vi "CRYSet SoundCard Front Panel.vi"(11 "Vi Ref in":refnum<vi> caption="Vi Ref") -> (3 "Vi Ref out":refnum<vi> caption="Vi Ref")   [LabVIEW 2013]
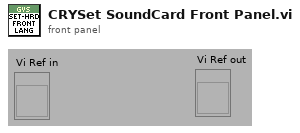
[diagram p1: front panel]
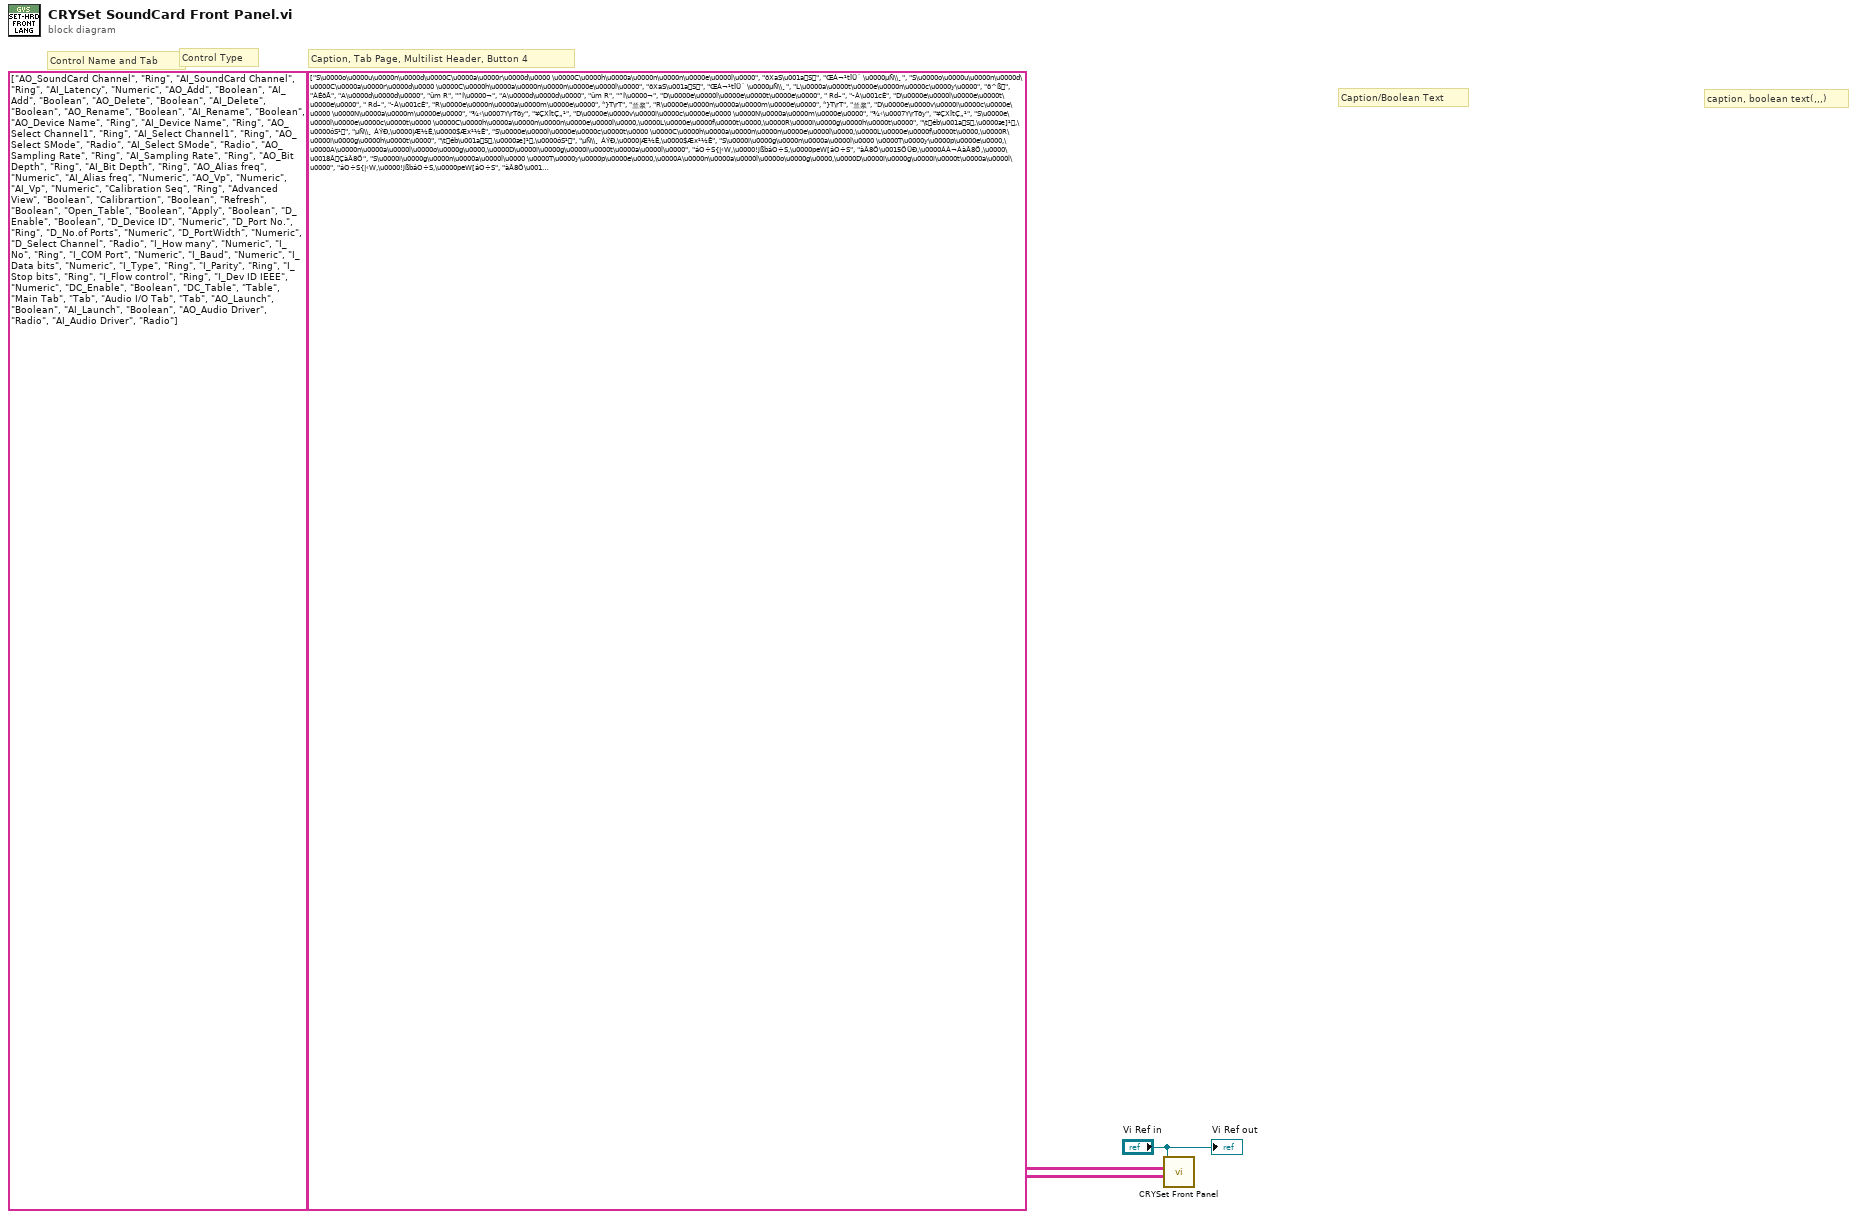
[diagram p0: block diagram]
diagram:
  # "Caption, Tab Page, Multilist Header, Button 4"
  # "Control Type"
  # "Control Name and Tab"
  # "caption, boolean text(,,,)"
  # "Caption/Boolean Text"
  n1 = call "CRYSet Front Panel.vi"("Caption(Boolean Text)"=string[][] [["S\u0000o\u0000u\u0000n\u0000d\u0000C\u0000a\u0000r\u0000d\u0000 \u0000C\u0000h\u0000a\u0000n\u0000n\u0000e\u0000l\u0000", "ðXaS\u001aS", "ŒÁ¬¹tÎÜ´ \u0000µÑ\\¸"], ["S\u0000o\u0000u\u0000n\u0000d\u0000C\u0000a\u0000r\u0000d\u0000 \u0000C\u0000h\u0000a\u0000n\u0000n\u0000e\u0000l\u0000", "ðXaS\u001aS", "ŒÁ¬¹tÎÜ´ \u0000µÑ\\¸"], ["L\u0000a\u0000t\u0000e\u0000n\u0000c\u0000y\u0000", "ö^ß", "ÀÉðÅ"], ["A\u0000d\u0000d\u0000", "ûm R", "”Í\u0000¬"], ["A\u0000d\u0000d\u0000", "ûm R", "”Í\u0000¬"], ["D\u0000e\u0000l\u0000e\u0000t\u0000e\u0000", " Rd–", "­À\u001cÈ"], ["D\u0000e\u0000l\u0000e\u0000t\u0000e\u0000", " Rd–", "­À\u001cÈ"], ["R\u0000e\u0000n\u0000a\u0000m\u0000e\u0000", "͑}T\rT", "兰浆"], ["R\u0000e\u0000n\u0000a\u0000m\u0000e\u0000", "͑}T\rT", "兰浆"], ["D\u0000e\u0000v\u0000i\u0000c\u0000e\u0000 \u0000N\u0000a\u0000m\u0000e\u0000", "¾‹\u0007Y\rTðy", "¥ÇXÎtÇ„¹"], ["D\u0000e\u0000v\u0000i\u0000c\u0000e\u0000 \u0000N\u0000a\u0000m\u0000e\u0000", "¾‹\u0007Y\rTðy", "¥ÇXÎtÇ„¹"], ["S\u0000e\u0000l\u0000e\u0000c\u0000t\u0000 \u0000C\u0000h\u0000a\u0000n\u0000n\u0000e\u0000l\u0000,\u0000L\u0000e\u0000f\u0000t\u0000,\u0000R\u0000i\u0000g\u0000h\u0000t\u0000", "\téb\u001aS,\u0000æ]¹,\u0000óS¹", "µÑ\\¸ ÁÝÐ,\u0000|Æ½Ê,\u0000$Æx¹½Ê"], ["S\u0000e\u0000l\u0000e\u0000c\u0000t\u0000 \u0000C\u0000h\u0000a\u0000n\u0000n\u0000e\u0000l\u0000,\u0000L\u0000e\u0000f\u0000t\u0000,\u0000R\u0000i\u0000g\u0000h\u0000t\u0000", "\téb\u001aS,\u0000æ]¹,\u0000óS¹", "µÑ\\¸ ÁÝÐ,\u0000|Æ½Ê,\u0000$Æx¹½Ê"], ["S\u0000i\u0000g\u0000n\u0000a\u0000l\u0000 \u0000T\u0000y\u0000p\u0000e\u0000,\u0000A\u0000n\u0000a\u0000l\u0000o\u0000g\u0000,\u0000D\u0000i\u0000g\u0000i\u0000t\u0000a\u0000l\u0000", "áO÷S{|‹W,\u0000!jßbáO÷S,\u0000peW[áO÷S", "àÂ8Ö\u0015ÖÜÐ,\u0000ÁÀ¬ÀàÂ8Ö,\u0000\u0018ÂÇàÂ8Ö"], ["S\u0000i\u0000g\u0000n\u0000a\u0000l\u0000 \u0000T\u0000y\u0000p\u0000e\u0000,\u0000A\u0000n\u0000a\u0000l\u0000o\u0000g\u0000,\u0000D\u0000i\u0000g\u0000i\u0000t\u0000a\u0000l\u0000", "áO÷S{|‹W,\u0000!jßbáO÷S,\u0000peW[áO÷S", "àÂ8Ö\u0015ÖÜÐ,\u0000ÁÀ¬ÀàÂ8Ö,\u0000\u0018ÂÇàÂ8Ö"], ["S\u0000a\u0000m\u0000p\u0000l\u0000i\u0000n\u0000g\u0000 \u0000R\u0000a\u0000t\u0000e\u0000", "Ç‘7h‡s", "\\Ôø¼TÖüÈ\fÓ\u0018Â"], ["S\u0000a\u0000m\u0000p\u0000l\u0000i\u0000n\u0000g\u0000 \u0000R\u0000a\u0000t\u0000e\u0000", "Ç‘7h‡s", "\\Ôø¼TÖüÈ\fÓ\u0018Â"], ["B\u0000i\u0000t\u0000 \u0000D\u0000e\u0000p\u0000t\u0000h\u0000", "Ôkyrpe", "É·ÇTÖD¾¸Ò\u0018Â"], ["B\u0000i\u0000t\u0000 \u0000D\u0000e\u0000p\u0000t\u0000h\u0000", "Ôkyrpe", "É·ÇTÖD¾¸Ò\u0018Â"], ["A\u0000l\u0000i\u0000a\u0000s\u0000 \u0000F\u0000r\u0000e\u0000e\u0000 \u0000F\u0000r\u0000e\u0000q\u0000(\u0000H\u0000z\u0000)\u0000", "\u0006Rgs\nNP", "ÈÕ\u0004ÇüÈ\fÓ\u0018Â"], ["A\u0000l\u0000i\u0000a\u0000s\u0000 \u0000F\u0000r\u0000e\u0000e\u0000 \u0000F\u0000r\u0000e\u0000q\u0000(\u0000H\u0000z\u0000)\u0000", "\u0006Rgs\nNP", "ÈÕ\u0004ÇüÈ\fÓ\u0018Â"], ["V\u0000p\u0000", "ð\\<P5u‹S\bÿV\u0000p\u0000\tÿ", "\u0004ÈUÅ(\u0000V\u0000p\u0000)\u0000"], ["V\u0000p\u0000", "ð\\<P5u‹S\bÿV\u0000p\u0000\tÿ", "\u0004ÈUÅ(\u0000V\u0000p\u0000)\u0000"], ["C\u0000a\u0000l\u0000i\u0000b\u0000r\u0000a\u0000t\u0000i\u0000o\u0000n\u0000 \u0000S\u0000e\u0000q\u0000u\u0000e\u0000n\u0000c\u0000e\u0000", "!hÆQ^\u0017R", "P­\u0000Éü¬\u001cÈ,¸"], ["A\u0000d\u0000v\u0000a\u0000n\u0000c\u0000e\u0000d\u0000 \u0000V\u0000i\u0000e\u0000w\u0000", "Ø§~\ty", "Ç8Á× \u0000ô¼0®"], ["C\u0000a\u0000l\u0000i\u0000b\u0000r\u0000a\u0000t\u0000i\u0000o\u0000n\u0000", "!hÆQ", "P­\u0000É"], ["R\u0000e\u0000f\u0000r\u0000e\u0000s\u0000h\u0000", "7R°elxöN", "¥ÇXÎ\u0015Èô¼ \u00001¬àÂ"], ["O\u0000p\u0000e\u0000n\u0000 \u0000T\u0000a\u0000b\u0000l\u0000e\u0000", "Sb\u0000_\u0017Rhˆ", "µÑ\\¸©º]¸"], ["A\u0000p\u0000p\u0000l\u0000y\u0000", "”^(u", "\u0001È©Æ"], ["E\u0000n\u0000a\u0000b\u0000l\u0000e\u0000", "/T(u", "\u0000¬¥²"], ["D\u0000e\u0000v\u0000i\u0000c\u0000e\u0000 \u0000I\u0000D\u0000", "¾‹\u0007Y\u0016÷S", "¥ÇXÎÝÂÄ¼ˆ¼8Ö\u0000"], ["P\u0000o\u0000r\u0000t\u0000 \u0000N\u0000o\u0000.\u0000", "ïzãS\u0016÷S", "ìÓl­ˆ¼8Ö"], ["N\u0000o\u0000.\u0000o\u0000f\u0000 \u0000P\u0000o\u0000r\u0000t\u0000s\u0000", "ïzãSpeÏ‘", "ìÓl­\u001c¬\u0018Â"], ["P\u0000o\u0000r\u0000t\u0000 \u0000W\u0000i\u0000d\u0000t\u0000h\u0000", "ïzãS½[¦^", "ìÓl­íÓ"], ["S\u0000e\u0000l\u0000e\u0000c\u0000t\u0000 \u0000C\u0000h\u0000a\u0000n\u0000n\u0000e\u0000l\u0000,\u0000O\u0000u\u0000t\u0000p\u0000u\u0000t\u0000,\u0000I\u0000n\u0000p\u0000u\u0000t\u0000", "\téb\u001aS,\u0000úQ,\u0000eQ", "µÑ\\¸ ÁÝÐ,\u0000œÍl­,\u0000…Çl­"], ["H\u0000o\u0000w\u0000 \u0000m\u0000a\u0000n\u0000y\u0000?\u0000", "¥cãSpeÏ‘", "‡º\u001c¬…ÇÈ²L®?\u0000"], ["I\u0000n\u0000t\u0000e\u0000r\u0000f\u0000a\u0000c\u0000e\u0000.\u0000N\u0000o", "¥cãS÷S", "\u0000³tºˆ¼8Ö"], ["C\u0000O\u0000M\u0000 \u0000P\u0000o\u0000r\u0000t\u0000", "2NL\u001a¯ïzãS", "C\u0000O\u0000M\u0000ìÓl­"], ["B\u0000a\u0000u\u0000d\u0000 \u0000R\u0000a\u0000t\u0000e\u0000", "âlyr‡s", "ô¼Ü´ÁÄ³"], ["D\u0000a\u0000t\u0000a\u0000 \u0000b\u0000i\u0000t\u0000s\u0000", "pencMO", "ÇÌ¸D¾¸Ò\u0018Â"], ["T\u0000y\u0000p\u0000e\u0000", "{|‹W", "\u0015Ö"], ["P\u0000a\u0000r\u0000i\u0000t\u0000y\u0000", "GYvP'`", "0®°Æ1Á"], ["S\u0000t\u0000o\u0000p\u0000 \u0000b\u0000i\u0000t\u0000s\u0000", "\\PbkMO", "\u0015ÈÀÉD¾¸Ò"], ["F\u0000l\u0000o\u0000w\u0000 \u0000c\u0000o\u0000n\u0000t\u0000r\u0000o\u0000l\u0000", "Am§c6R", "ÇÌ¸P×¹pÈÈ"], ["D\u0000e\u0000v\u0000 \u0000I\u0000D\u0000 \u0000I\u0000E\u0000E\u0000E\u0000", "緥\u0007Y\u0007h茓 \u0000I\u0000E\u0000E\u0000E\u0000", "¥ÇXÎˆ¼8Ö \u0000I\u0000E\u0000E\u0000E\u0000"], ["E\u0000n\u0000a\u0000b\u0000l\u0000e\u0000", "Oý€", "\u0000¬¥²"], ["T\u0000a\u0000b\u0000l\u0000e\u0000", "hˆ", "\\Ô"], ["S\u0000o\u0000u\u0000n\u0000d\u0000C\u0000a\u0000r\u0000d\u0000,\u0000D\u0000i\u0000g\u0000i\u0000t\u0000a\u0000l\u0000 \u0000I\u0000/\u0000O\u0000,\u0000I\u0000n\u0000t\u0000e\u0000r\u0000f\u0000a\u0000c\u0000e\u0000,\u0000H\u0000e\u0000l\u0000p\u0000", "ðXaS,\u0000peW[ \u0000I\u0000/\u0000O\u0000,\u0000¥cãS,\u0000.^©R \u0000", "LÇ1Á,\u0000\u0018ÂÇÇÍl­,\u0000\u0000³tº,\u0000Ä³ÀÆÐ¹"], ["O\u0000u\u0000t\u0000p\u0000u\u0000t\u0000,\u0000I\u0000n\u0000p\u0000u\u0000t\u0000", "úQ,\u0000eQ", "œÍl­,\u0000…Çl­"], ["A\u0000S\u0000I\u0000O\u0000 \u0000C\u0000o\u0000n\u0000t\u0000r\u0000o\u0000l\u0000 \u0000P\u0000a\u0000n\u0000e\u0000l\u0000", "A\u0000S\u0000I\u0000O\u0000§c6Rb—g", "A\u0000S\u0000I\u0000O\u0000 \u0000pÈ…È\u0010Ó"], ["A\u0000S\u0000I\u0000O\u0000 \u0000C\u0000o\u0000n\u0000t\u0000r\u0000o\u0000l\u0000 \u0000P\u0000a\u0000n\u0000e\u0000l\u0000", "A\u0000S\u0000I\u0000O\u0000§c6Rb—g", "A\u0000S\u0000I\u0000O\u0000 \u0000pÈ…È\u0010Ó"], ["A\u0000u\u0000d\u0000i\u0000o\u0000 \u0000D\u0000r\u0000i\u0000v\u0000e\u0000r\u0000,\u0000W\u0000D\u0000M\u0000/\u0000M\u0000M\u0000E\u0000,\u0000A\u0000S\u0000I\u0000O\u0000", "ðXaSqš¨R,\u0000W\u0000D\u0000M\u0000/\u0000M\u0000M\u0000E\u0000,\u0000A\u0000S\u0000I\u0000O\u0000", "A\u0000u\u0000d\u0000i\u0000o\u0000 \u0000D\u0000r\u0000i\u0000v\u0000e\u0000r\u0000,\u0000W\u0000D\u0000M\u0000/\u0000M\u0000M\u0000E\u0000,\u0000A\u0000S\u0000I\u0000O\u0000"], ["A\u0000u\u0000d\u0000i\u0000o\u0000 \u0000D\u0000r\u0000i\u0000v\u0000e\u0000r\u0000,\u0000W\u0000D\u0000M\u0000/\u0000M\u0000M\u0000E\u0000,\u0000A\u0000S\u0000I\u0000O\u0000", "ðXaSqš¨R,\u0000W\u0000D\u0000M\u0000/\u0000M\u0000M\u0000E\u0000,\u0000A\u0000S\u0000I\u0000O\u0000", "A\u0000u\u0000d\u0000i\u0000o\u0000 \u0000D\u0000r\u0000i\u0000v\u0000e\u0000r\u0000,\u0000W\u0000D\u0000M\u0000/\u0000M\u0000M\u0000E\u0000,\u0000A\u0000S\u0000I\u0000O\u0000"]], "Control ID and Type(Label Name, Type)"=string[][] [["AO_SoundCard Channel", "Ring"], ["AI_SoundCard Channel", "Ring"], ["AI_Latency", "Numeric"], ["AO_Add", "Boolean"], ["AI_Add", "Boolean"], ["AO_Delete", "Boolean"], ["AI_Delete", "Boolean"], ["AO_Rename", "Boolean"], ["AI_Rename", "Boolean"], ["AO_Device Name", "Ring"], ["AI_Device Name", "Ring"], ["AO_Select Channel1", "Ring"], ["AI_Select Channel1", "Ring"], ["AO_Select SMode", "Radio"], ["AI_Select SMode", "Radio"], ["AO_Sampling Rate", "Ring"], ["AI_Sampling Rate", "Ring"], ["AO_Bit Depth", "Ring"], ["AI_Bit Depth", "Ring"], ["AO_Alias freq", "Numeric"], ["AI_Alias freq", "Numeric"], ["AO_Vp", "Numeric"], ["AI_Vp", "Numeric"], ["Calibration Seq", "Ring"], ["Advanced View", "Boolean"], ["Calibrartion", "Boolean"], ["Refresh", "Boolean"], ["Open_Table", "Boolean"], ["Apply", "Boolean"], ["D_Enable", "Boolean"], ["D_Device ID", "Numeric"], ["D_Port No.", "Ring"], ["D_No.of Ports", "Numeric"], ["D_PortWidth", "Numeric"], ["D_Select Channel", "Radio"], ["I_How many", "Numeric"], ["I_No", "Ring"], ["I_COM Port", "Numeric"], ["I_Baud", "Numeric"], ["I_Data bits", "Numeric"], ["I_Type", "Ring"], ["I_Parity", "Ring"], ["I_Stop bits", "Ring"], ["I_Flow control", "Ring"], ["I_Dev ID IEEE", "Numeric"], ["DC_Enable", "Boolean"], ["DC_Table", "Table"], ["Main Tab", "Tab"], ["Audio I/O Tab", "Tab"], ["AO_Launch", "Boolean"], ["AI_Launch", "Boolean"], ["AO_Audio Driver", "Radio"], ["AI_Audio Driver", "Radio"]], "Vi Ref"="Vi Ref in") -> ()  [unwired: 9 in]
  "Vi Ref out" <- "Vi Ref in"
